vi "CAN_ReadBoardInfo.vi"(8 "错误输入（无错误）":errorcluster, 11 "General_Input":T1={"DevType"=1, "DevIndex"=0, "CANIndex"=0} {"CANIndex" items=["0", "1"]; "DevType" items=["PCI5121"=1, "PCI9810"=2, "USBCAN1"=3, "USBCAN2"=4, "PCI9820"=5, "CAN232"=6, "PCI5110"=7, "CANLite(mini)"=8, "ISA9620"=9, "ISA5420"=10, "PC104CAN"=11, "CANETE"=12, "DNP9810"=13, "PCI9840B"=14, "PC104C2"=15, "PCI9820I"=16]}) -> (0 "错误输出":errorcluster, 2 "VCI_BOARD_INFO":T2 {"in_Version" format="%x"; "dr_Version" format="%x"; "fw_Version" format="%x"; "hw_Version" format="%x"}, 3 "General_Output":T1={"DevType"=1, "DevIndex"=0, "CANIndex"=0} {"CANIndex" items=["0", "1"]; "DevType" items=["PCI5121"=1, "PCI9810"=2, "USBCAN1"=3, "USBCAN2"=4, "PCI9820"=5, "CAN232"=6, "PCI5110"=7, "CANLite(mini)"=8, "ISA9620"=9, "ISA5420"=10, "PC104CAN"=11, "CANETE"=12, "DNP9810"=13, "PCI9840B"=14, "PC104C2"=15, "PCI9820I"=16]})   [LabVIEW 2012]
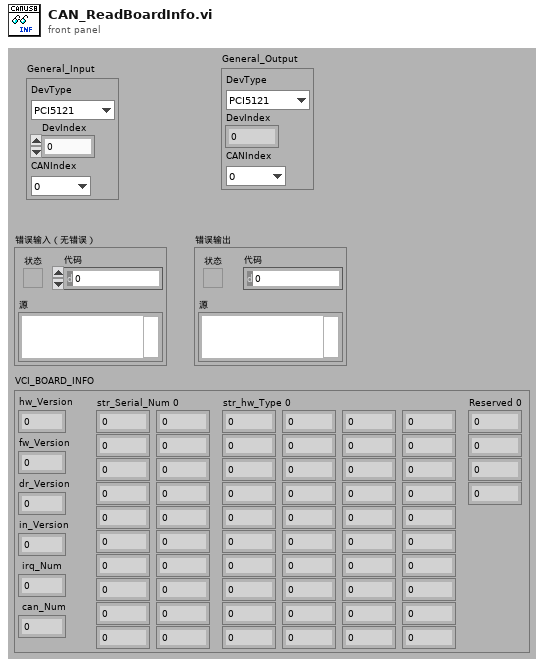
[diagram p1: front panel]
types:
  T1 = cluster{"DevType":u16, "DevIndex":u32, "CANIndex":u16}
  T2 = cluster{"hw_Version":u16, "fw_Version":u16, "dr_Version":u16, "in_Version":u16, "irq_Num":u16, "can_Num":u8, "str_Serial_Num 0":i8, "str_Serial_Num 1":i8, "str_Serial_Num 2":i8, "str_Serial_Num 3":i8, "str_Serial_Num 4":i8, "str_Serial_Num 5":i8, "str_Serial_Num 6":i8, "str_Serial_Num 7":i8, "str_Serial_Num 8":i8, "str_Serial_Num 9":i8, "str_Serial_Num 10":i8, "str_Serial_Num 11":i8, "str_Serial_Num 12":i8, "str_Serial_Num 13":i8, "str_Serial_Num 14":i8, "str_Serial_Num 15":i8, "str_Serial_Num 16":i8, "str_Serial_Num 17":i8, "str_Serial_Num 18":i8, "str_Serial_Num 19":i8, "str_hw_Type 0":i8, "str_hw_Type 1":i8, "str_hw_Type 2":i8, "str_hw_Type 3":i8, "str_hw_Type 4":i8, "str_hw_Type 5":i8, "str_hw_Type 6":i8, "str_hw_Type 7":i8, "str_hw_Type 8":i8, "str_hw_Type 9":i8, "str_hw_Type 10":i8, "str_hw_Type 11":i8, "str_hw_Type 12":i8, "str_hw_Type 13":i8, "str_hw_Type 14":i8, "str_hw_Type 15":i8, "str_hw_Type 16":i8, "str_hw_Type 17":i8, "str_hw_Type 18":i8, "str_hw_Type 19":i8, "str_hw_Type 20":i8, "str_hw_Type 21":i8, "str_hw_Type 22":i8, "str_hw_Type 23":i8, "str_hw_Type 24":i8, "str_hw_Type 25":i8, "str_hw_Type 26":i8, "str_hw_Type 27":i8, "str_hw_Type 28":i8, "str_hw_Type 29":i8, "str_hw_Type 30":i8, "str_hw_Type 31":i8, "str_hw_Type 32":i8, "str_hw_Type 33":i8, "str_hw_Type 34":i8, "str_hw_Type 35":i8, "str_hw_Type 36":i8, "str_hw_Type 37":i8, "str_hw_Type 38":i8, "str_hw_Type 39":i8, "Reserved 0":dbl, "Reserved 1":dbl, "Reserved 2":dbl, "Reserved 3":dbl}
  T3 = cluster{"DeviceType":u32, "DeviceIndex":u32, "CANIndex":u16}
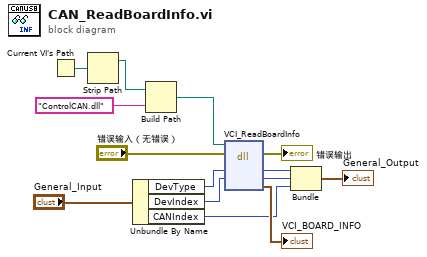
[diagram p0: block diagram]
diagram:
  n1 = Current VI's Path() -> (path=w9:path)
  n2 = Strip Path(path=w9) -> (stripped path=w10:path)  [unwired: 1 out]
  n3 = Unbundle By Name("General_Input") -> ("DevType"=w7:u16, "DevIndex"=w6:u32, "CANIndex"=w2:u16)
  n4 = Build Path(base path=w10, name or relative path="ControlCAN.dll" ("名称或相对路径")) -> (appended path=w5:path)
  n5 = dll-call lib="E:/1_Projects/ITMS/API Library/ControlCAN.dll" fn="VCI_ReadBoardInfo"(path in=w5, error in="错误输入（无错误）", "DeviceType"=w7, "DeviceIndex"=w6) -> (error out=→"错误输出":errorcluster, "DeviceType"=w4:u32, "DeviceIndex"=w3:u32, "VCI_BOARD_INFO"=→"VCI_BOARD_INFO":T2)  [unwired: 3 in, 1 out]
  n6 = Bundle("DeviceType"=w4, "DeviceIndex"=w3, "CANIndex"=w2) -> (→"General_Output":T3)  [unwired: 1 in]
